vi "set_done_flag.vi"(8 "error in (no error)":errorcluster, 10 "done?":bool, 11 "GenericSweep in":refnum<class "GenericSweep.lvclass">) -> (0 "error out":errorcluster, 3 "GenericSweep out":refnum<class "GenericSweep.lvclass">)   [LabVIEW 2010, in "GenericSweep.lvclass"]
uses:
  GenericSweep.lvclass
  GenericSweep.lvclass/GenericSweep.ctl
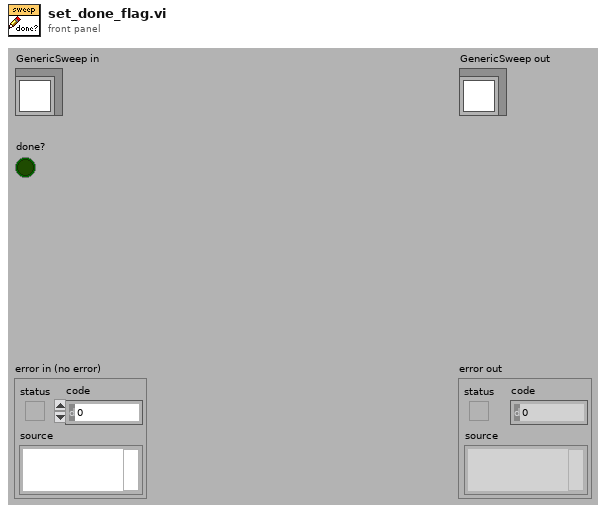
[diagram p1: front panel]
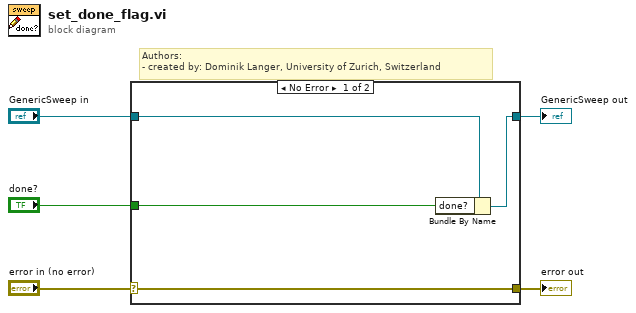
[diagram p0: block diagram]
diagram:
  # "Authors: \n- created by: Dominik Langer, University of Zurich, Switzerland"
  n1 = case shown="No Error" "error in (no error)" {
    selector: "error in (no error)" -> [w9 w10]
    tunnel: [w9 w10] -> w4
    tunnel: [w7 w11] -> w2
    tunnel: "GenericSweep in" -> [w8 w11]
    tunnel: "done?" -> [w6 _]
    frame No Error {
      n2 = Bundle By Name(cluster=w8, "done?"=w6) -> (w7:refnum<class "GenericSweep.lvclass">)
    }
    frame Error {
    }
  }
  "error out" <- w4
  "GenericSweep out" <- w2
